vi "accelerometer detector.vi"(0 "Calibration":T1, 1 "Data":sgl[][][](array[numeric]), 2 "1 accel found?":bool[](array[boolean]), 4 "Nº meas":i32) -> (7 "output cluster":T1, 8 "report":string, 9 "Continuar?":bool)   [LabVIEW 2015]
doc: "check that there are enough correct calibration files to continue"
uses:
  controls/Calibration Data.ctl
panel:
  out "Accel detected":i32
  out "max index(es)":i32
  out "max value":i32
  out "Array 3":i32[](array[numeric])
  out "sorted array":i32[](array[numeric])
  out "Array":i32[](array[numeric])
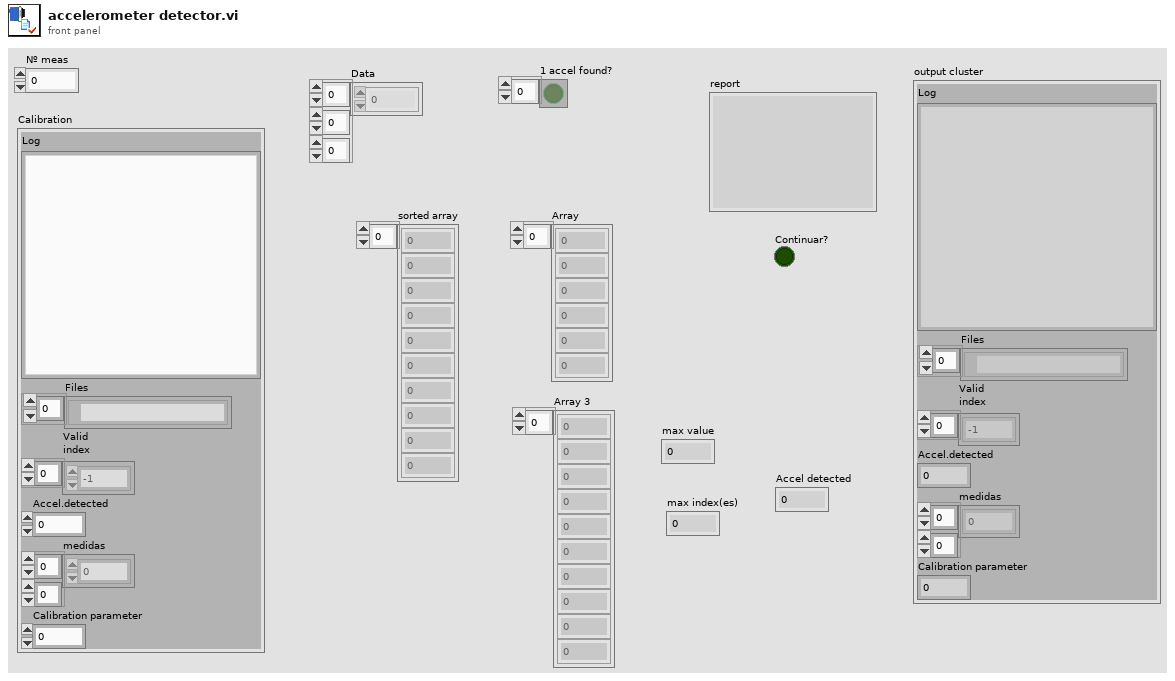
[diagram p1: front panel]
types:
  T1 = typedef "Calibration Data.ctl" = cluster{"Log":string, "Files":path[], "Valid\nindex":i32[], "Accel.detected":i32, "medidas":sgl[][], "Calibration parameter":dbl}
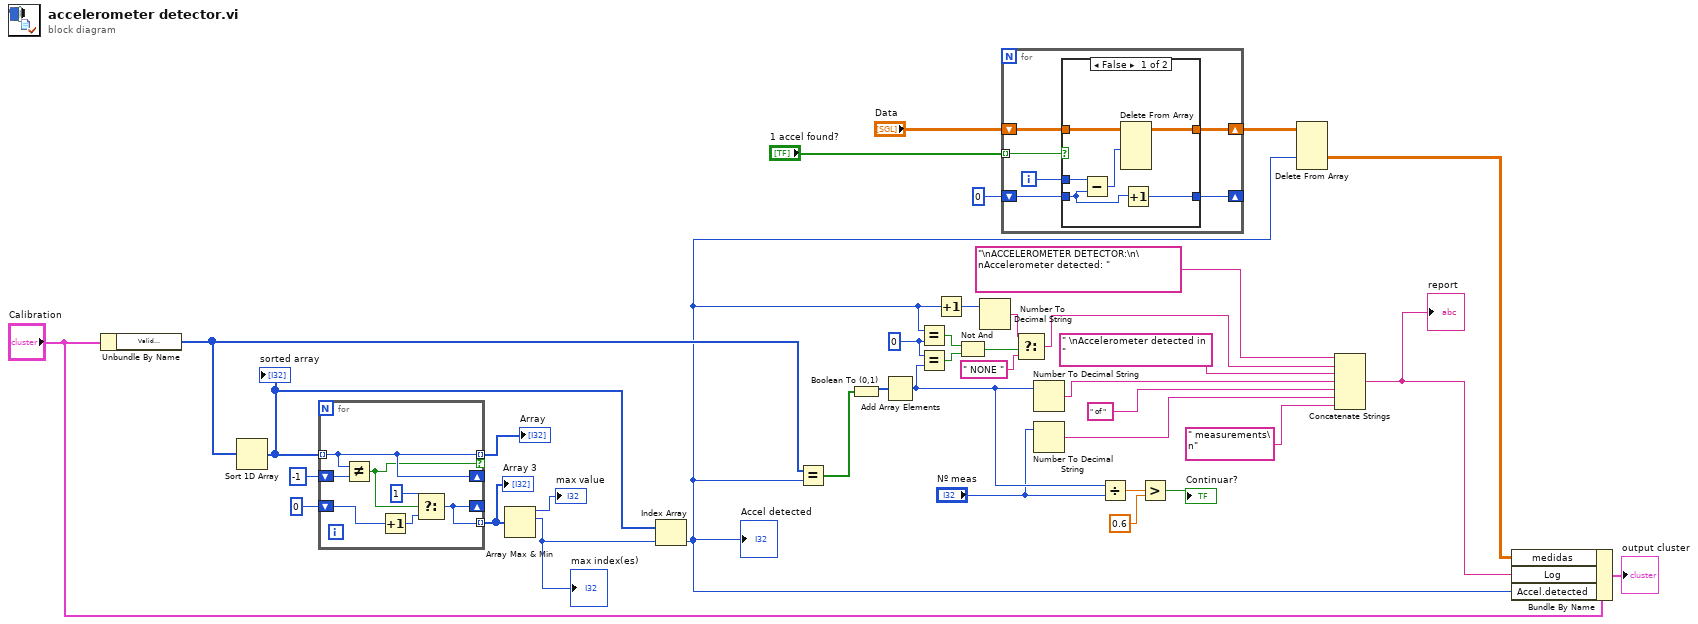
[diagram p0: block diagram]
diagram:
  w18 = 0 ("index of element")
  n1 = Unbundle By Name("Calibration") -> ("Valid\nindex"=w9:i32[])
  n2 = Sort 1D Array(array=w9) -> (sorted array=w19:i32[])
  "sorted array" <- w19
  n3 = for {
    tunnel: w19 -> [w44] mode=indexing
    shift-right: [w44] -> _
    shift-left: -1 ("y") -> [w45]
    tunnel: [w44] -> w27 mode=indexing if=w43
    shift-right: [w40] -> _
    shift-left: 0 ("y") -> [w41]
    tunnel: [w40] -> w25 mode=indexing
    n4 = Not Equal?(x=w44, y=w45) -> (x != y?=w43:bool)
    n5 = Increment(x=w41) -> (x+1=w42:i32)
    n6 = Select(t=1 ("y"), s=w43, f=w42) -> (s? t:f=w40:i32)
  }
  "Array" <- w27
  "Array 3" <- w25
  n7 = Array Max & Min(array=w25) -> (max value=→"max value":i32, max index (indices)=w23:i32)  [unwired: 2 out]
  "max index(es)" <- w23
  n8 = Index Array(array=w19, index=w23) -> (element=w6:i32)
  "Accel detected" <- w6
  n9 = Equal?(x=w9, y=w6) -> (x = y?=w21:bool[])
  n10 = Boolean To (0,1)(Boolean=w21) -> (0, 1=w20:i16[])
  n11 = Add Array Elements(numeric array=w20) -> (sum=w13:i16)
  n12 = Equal?(x=w6, y=w18) -> (x = y?=w16:bool)
  n13 = Equal?(x=w18, y=w13) -> (x = y?=w15:bool)
  n14 = Increment(x=w6) -> (x+1=w22:i32)
  n15 = Not And(1:w15, 2:w16) -> (0:w14:bool)
  n16 = Number To Decimal String(number=w22) -> (decimal integer string=w11:string)  [unwired: 1 in]
  n17 = for {
    tunnel: "1 accel found?" -> [w50] mode=indexing
    shift-right: [w49] -> w35
    shift-left: "Data" -> [w51]
    shift-right: [w46] -> _
    shift-left: 0 ("index of element") -> [w47]
    i -> [w48]
    n18 = case shown="False" w50 {
      tunnel: w51 -> [w57 w59]
      tunnel: [w56 w59] -> w49
      tunnel: w48 -> [w55 _]
      tunnel: w47 -> [w52 w58]
      tunnel: [w53 w58] -> w46
      frame False {
        n19 = Subtract(x=w55, y=w52) -> (x-y=w54:i32)
        n20 = Delete From Array(array=w57, index (dim 0)=w54) -> (array with subset deleted=w56:sgl[][][])  [unwired: 3 in, 1 out]
        n21 = Increment(x=w52) -> (x+1=w53:i32)
      }
      frame True {
      }
    }
  }
  n22 = Select(t=w11, s=w14, f=" NONE ") -> (s? t:f=w12:string)
  n23 = Number To Decimal String(number=w13) -> (decimal integer string=w38:string)  [unwired: 1 in]
  n24 = Number To Decimal String(number="Nº meas") -> (decimal integer string=w36:string)  [unwired: 1 in]
  n25 = Divide(x=w13, y="Nº meas") -> (x/y=w33:dbl)
  n26 = Greater?(x=w33, y=0.6) -> (0:→"Continuar?":bool)
  n27 = Delete From Array(array=w35, index (dim 1)=w6) -> (deleted portion=w4:sgl[][])  [unwired: 3 in, 1 out]
  n28 = Concatenate Strings("\nACCELEROMETER DETECTOR:\n\nAccelerometer detected: ", w12, " \nAccelerometer detected in  ", w38, " of ", w36, " measurements\n") -> (w1:string)
  "report" <- w1
  n29 = Bundle By Name(cluster="Calibration", "medidas"=w4, "Log"=w1, "Accel.detected"=w6) -> (→"output cluster":T1)
